vi "Close App Ref.vi"(0 "LV DEV in":refnum<class "LV DEV.lvclass">, 11 "error in (no error)":errorcluster) -> (4 "LV DEV out":refnum<class "LV DEV.lvclass">, 15 "error out":errorcluster)   [LabVIEW 2016, in "LV DEV.lvclass"]
uses:
  LV DEV.lvclass
  LV DEV.lvclass/LV DEV.ctl
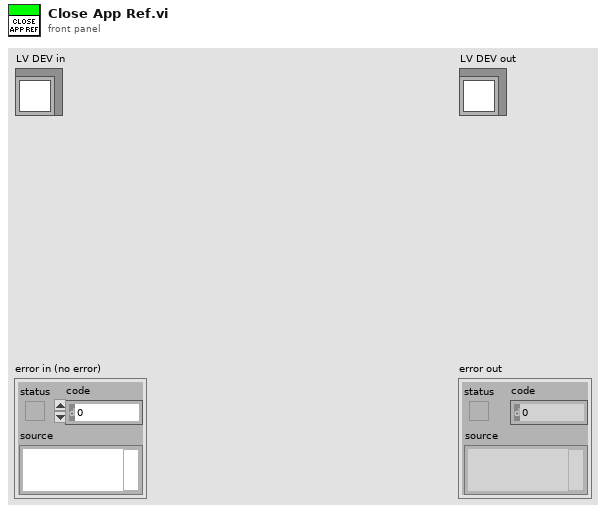
[diagram p1: front panel]
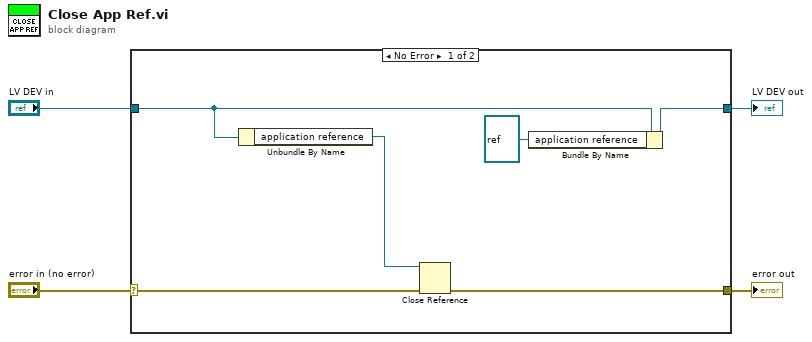
[diagram p0: block diagram]
diagram:
  n1 = case shown="No Error" "error in (no error)" {
    selector: "error in (no error)" -> [w10 w12]
    tunnel: [w9 w12] -> w3
    tunnel: [w6 w11] -> w1
    tunnel: "LV DEV in" -> [w7 w11]
    frame No Error {
      n2 = Unbundle By Name(w7) -> ("application reference"=w8:refnum<vi>)
      n3 = Close Reference(reference=w8, error in (no error)=w10) -> (error out=w9:errorcluster)
      n4 = Bundle By Name(cluster=w7, "application reference"=refnum<vi> refnum) -> (w6:refnum<class "LV DEV.lvclass">)
    }
    frame Error {
    }
  }
  "error out" <- w3
  "LV DEV out" <- w1
